vi "test_GetItemInfosFromProjectFile_VersionSampleProject.vi"() -> (3 "Pass?":bool)   [LabVIEW 2019, in "Tests.SolutionBuilder.lvlib"]
uses:
  Tests.SolutionBuilder.lvlib
  SolutionBuilder/SolutionBuilder.lvclass
  SolutionBuilder/SolutionBuilder.lvclass/SolutionBuilder.ctl
  SolutionBuilder/ProjectItem/ProjectItem.lvclass/ProjectItem.ctl
  SolutionBuilder/ProjectItem/ProjectItem.lvclass
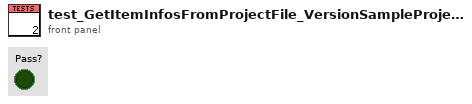
[diagram p1: front panel]
types:
  T1 = typedef "SolutionBuilder.lvlib/SolutionBuilder.lvclass/ProjectItemMap.ctl" = map{path, refnum<class "ProjectItem.lvclass">[]}
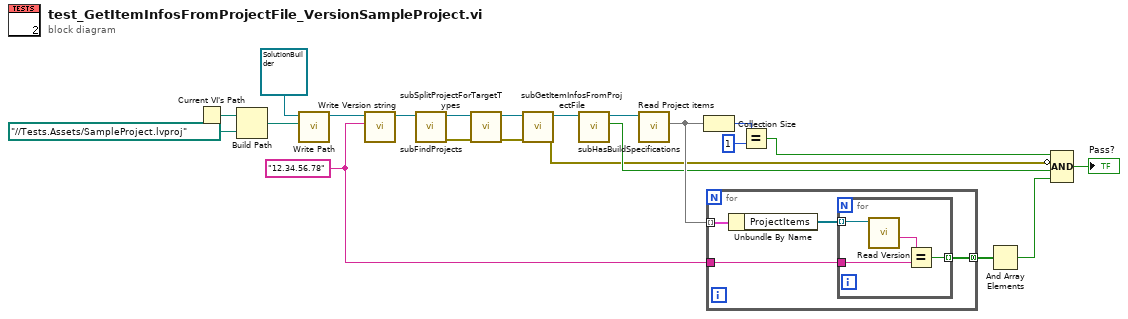
[diagram p0: block diagram]
diagram:
  w4 = "12.34.56.78" ("Version string")
  n1 = Current VI's Path() -> (path=w21:path)
  n2 = Build Path(base path=w21, name or relative path=path "../../Tests.Assets/SampleProject.lvproj" ("Path")) -> (appended path=w19:path)
  n3 = call "Write Path.vi"("Path"=w19, "SolutionBuilder in"=refnum<class "SolutionBuilder.lvclass"> refnum) -> ("SolutionBuilder out"=w6:refnum<class "SolutionBuilder.lvclass">)  [unwired: 9 in]
  n4 = call "Write Version string.vi"("Version string"=w4, "SolutionBuilder in"=w6) -> ("SolutionBuilder out"=w5:refnum<class "SolutionBuilder.lvclass">)  [unwired: 9 in]
  n5 = call "subFindProjects.vi"("SolutionBuilder in"=w5) -> ("error out"=w10:errorcluster, "SolutionBuilder out"=w11:refnum<class "SolutionBuilder.lvclass">)  [unwired: 9 in]
  n6 = call "subSplitProjectForTargetTypes.vi"("error in (no error)"=w10, "SolutionBuilder in"=w11) -> ("error out"=w9:errorcluster, "SolutionBuilder out"=w8:refnum<class "SolutionBuilder.lvclass">)  [unwired: 8 in]
  n7 = call "subGetItemInfosFromProjectFile.vi"("error in (no error)"=w9, "SolutionBuilder in"=w8) -> ("error out"=w13:errorcluster, "SolutionBuilder out"=w7:refnum<class "SolutionBuilder.lvclass">)  [unwired: 8 in]
  n8 = call "subHasBuildSpecifications.vi"("SolutionBuilder in"=w7) -> ("Has specs?"=w14:bool, "SolutionBuilder out"=w15:refnum<class "SolutionBuilder.lvclass">)  [unwired: 8 in, 1 out]
  n9 = call "Read Project items.vi"("SolutionBuilder in"=w15) -> ("Project items"=w16:T1)  [unwired: 9 in, 1 out]
  n10 = Collection Size(1:w16) -> (0:w18:i32)
  n11 = for {
    tunnel: w16 -> [w26] mode=indexing
    tunnel: w4 -> [w24]
    tunnel: [w23] -> w3 mode=concatenating
    n12 = Unbundle By Name(w26) -> ("ProjectItems"=w25:refnum<class "ProjectItem.lvclass">[])
    n13 = for {
      tunnel: w25 -> [w30] mode=indexing
      tunnel: w24 -> [w28]
      tunnel: [w27] -> w23 mode=indexing
      n14 = call "Read Version.vi"("ProjectItem in"=w30) -> ("Version string"=w29:string)  [unwired: 8 in, 2 out]
      n15 = Equal?(x=w29, y=w28) -> (x = y?=w27:bool)
    }
  }
  n16 = Equal?(x=w18, y=1) -> (x = y?=w1:bool)
  n17 = And Array Elements(Boolean array=w3) -> (logical AND=w2:bool)
  n18 = Compound Arithmetic op=AND(w1, invert w13, w14, w2) -> (→"Pass?":bool)
